vi "CANArry2Bits.vi"(0 "重构的Data数组输入":u32[][](array[numeric]), 5 "CAN_ID":string, 7 "Signal":string, 9 "Style":string, 12 "mpor":string[](array[string])) -> (2 "报文数量":i32, 3 "筛选的报文数组":u32[][](array[numeric]), 8 "CAN64B簇":cluster{"时间(s)":dbl[], "Data64Bits(u64)":u64[]})   [LabVIEW 2015]
panel:
  in  "ClusterSigFormat":T1
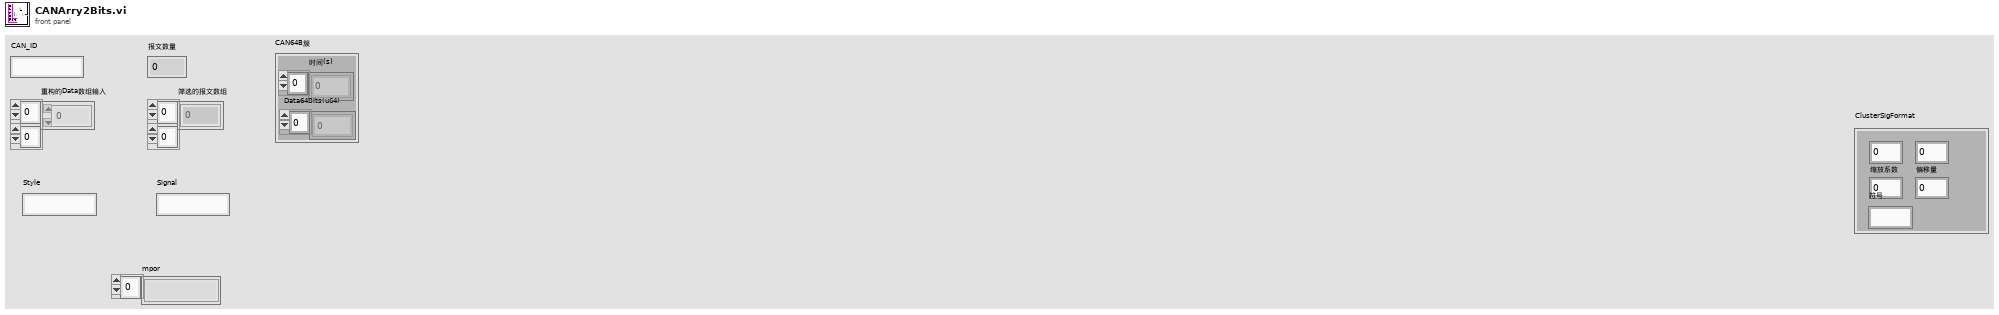
[diagram p1: front panel]
types:
  T1 = cluster{"起始位":u8, "长度":u8, "缩放系数":dbl, "偏移量":dbl, "符号":string}
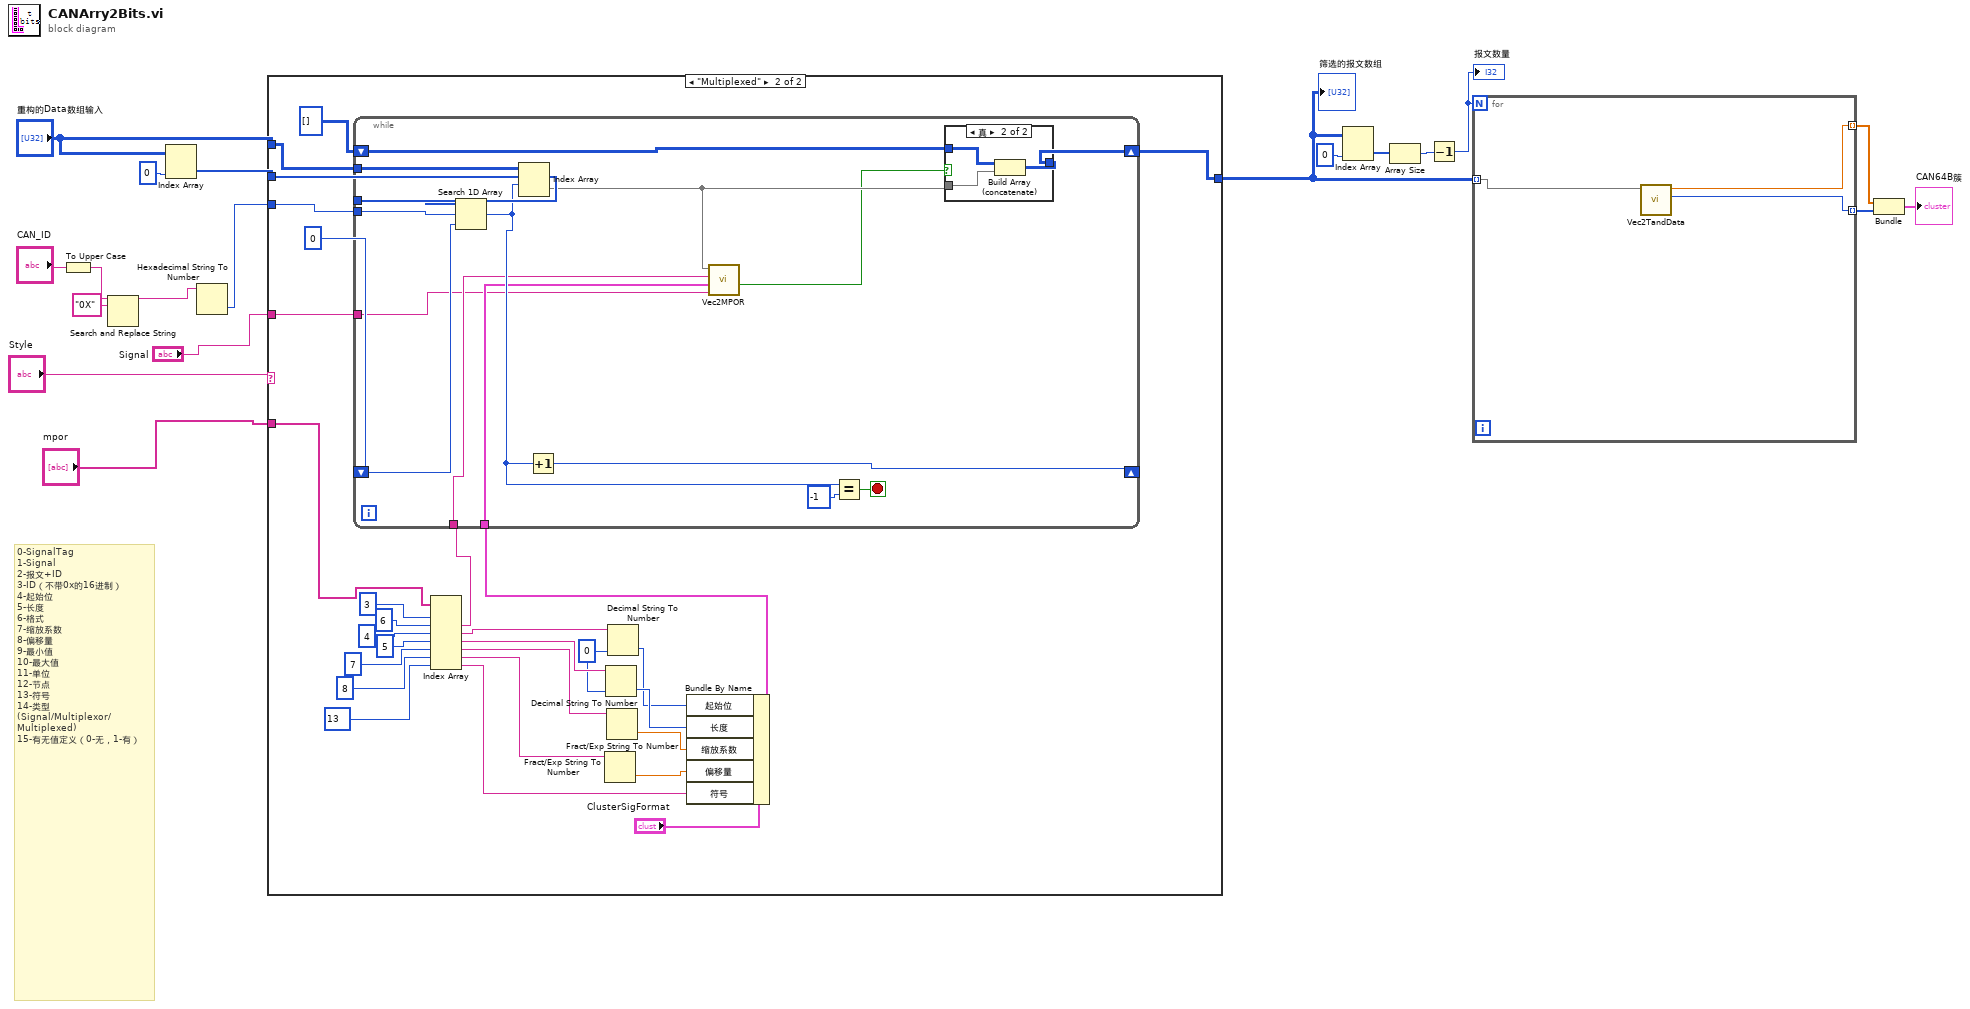
[diagram p0: block diagram]
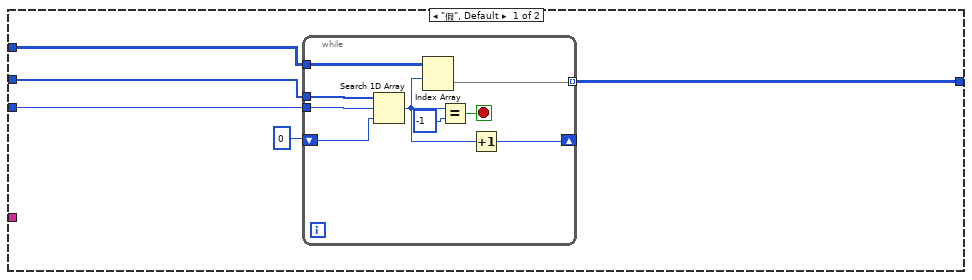
[diagram p2: hidden frame]
diagram:
  # "0-SignalTag\n1-Signal\n2-报文+ID\n3-ID（不带0x的16进制）\n4-起始位\n5-长度\n6-格式\n7-缩放系数\n8-偏移量\n9-最小值\n10-最大值\n11-单位\n12-节点\n13-符号\n14-类型\n(Signal/Multiplexor/\nMultiplexed)\n15-有无值定义（0-无，1-有）"
  n1 = To Upper Case(1:"CAN_ID") -> (0:w6:string)
  n2 = Search and Replace String(input string=w6, search string="0X" ("搜索字符串")) -> (result string=w4:string)  [unwired: 6 in, 3 out]
  n3 = Index Array(array="重构的Data数组输入", index (col)=0 ("禁用的索引 (列)")) -> (element=w15:u32[])  [unwired: 1 in]
  n4 = Hexadecimal String To Number(string=w4) -> (number=w14:u32)  [unwired: 2 in, 1 out]
  n5 = case shown="\"Multiplexed\"" "Style" {
    tunnel: [w24 w35] -> w18
    tunnel: "重构的Data数组输入" -> [w23 w61]
    tunnel: w15 -> [w21 w59]
    tunnel: w14 -> [w20 w58]
    tunnel: "mpor" -> [_ w39]
    tunnel: "Signal" -> [_ w34]
    frame "假", Default {
      n6 = while {
        tunnel: w21 -> [w33]
        tunnel: w20 -> [w31]
        tunnel: w23 -> [w30]
        tunnel: [w29] -> w24 mode=indexing
        shift-right: [w26] -> _
        shift-left: 0 -> [w32]
        stop <- w28 stop-if-true
        n7 = Search 1D Array(1D array=w33, element=w31, start index (0)=w32) -> (index of element=w25:i32)
        n8 = Index Array(array=w30, index (row)=w25) -> (element=w29:u32[])  [unwired: 1 in]
        n9 = Equal?(x=w25, y=-1) -> (x = y?=w28:bool)
        n10 = Increment(x=w25) -> (x+1=w26:i32)
      }
    }
    frame "Multiplexed" {
      w49 = u8 0 ("默认(0 I32)")
      n11 = Index Array(array=w39, index #1=3 ("索引"), index #2=6 ("索引"), index #3=4 ("索引"), index #4=5 ("索引"), index #5=7 ("索引"), index #6=8 ("索引"), index #7=13 ("索引")) -> (element #2=w38:string, element #3=w51:string, element #4=w50:string, element #5=w47:string, element #6=w48:string, element #7=w44:string)  [unwired: 1 out]
      n12 = Fract/Exp String To Number(string=w48) -> (number=w43:dbl)  [unwired: 3 in, 1 out]
      n13 = Decimal String To Number(string=w50, default (0L)=w49) -> (number=w41:u8)  [unwired: 1 in, 1 out]
      n14 = Fract/Exp String To Number(string=w47) -> (number=w42:dbl)  [unwired: 3 in, 1 out]
      n15 = Decimal String To Number(string=w51, default (0L)=w49) -> (number=w40:u8)  [unwired: 1 in, 1 out]
      n16 = Bundle By Name(cluster="ClusterSigFormat", "起始位"=w40, "长度"=w41, "缩放系数"=w42, "偏移量"=w43, "符号"=w44) -> (w37:T1)
      n17 = while {
        tunnel: w59 -> [w76]
        tunnel: w58 -> [w74]
        tunnel: w61 -> [w73]
        shift-right: [w70] -> _
        shift-left: 0 -> [w75]
        tunnel: w38 -> [w66]
        tunnel: w37 -> [w65]
        shift-right: [w68] -> w35
        shift-left: u32[][] [] ("重构的Data数组输入") -> [w67]
        tunnel: w34 -> [w63]
        stop <- w72 stop-if-true
        n18 = Search 1D Array(1D array=w76, element=w74, start index (0)=w75) -> (index of element=w69:i32)
        n19 = Index Array(array=w73, index (row)=w69) -> (element=w64:u32[])  [unwired: 1 in]
        n20 = Increment(x=w69) -> (x+1=w70:i32)
        n21 = call "Vec2MPOR.vi"("SignalName"=w63, "ClusterSigFormat"=w65, "格式"=w66, "DataIn"=w64) -> ("isTrue"=w62:bool)  [unwired: 6 in, 1 out]
        n22 = Equal?(x=w69, y=-1) -> (x = y?=w72:bool)
        n23 = case shown="真" w62 {
          tunnel: [w77 w80] -> w68
          tunnel: w67 -> [w77 w79]
          tunnel: w64 -> [_ w78]
          frame False {
          }
          frame True {
            n24 = Build Array (concatenate)(w79, w78) -> (w80:u32[][])
          }
        }
      }
    }
  }
  "筛选的报文数组" <- w18
  n25 = Index Array(array=w18, index (col)=0 ("禁用的索引 (列)")) -> (element=w11:u32[])  [unwired: 1 in]
  n26 = Array Size(array=w11) -> (size(s)=w13:i32)
  n27 = Decrement(x=w13) -> (x-1=w19:i32)
  "报文数量" <- w19
  n28 = for {
    N: w19 -> [_]
    tunnel: w18 -> [w81] mode=indexing
    tunnel: [w83] -> w10 mode=indexing
    tunnel: [w82] -> w9 mode=indexing
    n29 = call "Vec2TandData.vi"("Frames"=w81) -> ("_64Bits"=w82:u64, "时间(秒)"=w83:dbl)  [unwired: 9 in]
  }
  n30 = Bundle(w10, w9) -> (→"CAN64B簇":cluster{dbl[], u64[]})  [unwired: 1 in]
